vi "GVSGraph Main.vi"() -> ()   [LabVIEW 2013]
uses:
  Control/SplitterBar.ctl
  Control/Graph Main Info Cluster.ctl
  <vilib>/Utility/inputDevices.llb/closeMouse.vi
  GVSNew View Global.vi
  GVSView Global.vi
  <vilib>/Utility/inputDevices.llb/mouseAcquire.vi
  <vilib>/Utility/cursorutil.llb/Set Cursor (Icon Pict).vi
panel:
  in  "bWaitCommand":bool
  in  "Docking Start":bool
  in  "nIDV":i32=10
  in  "pSPRefParent":refnum<vi>
  in  "pVIRefParent":refnum<vi>
  in  "sViewName":string="DataView"
  out "Index":i32
  in  "stop":bool
  out "StateOut":bool
  out "Bar_shadow":bool
  in  "Resize FrontPanel":bool
  in  "Add Top":bool
  in  "Add Left":bool
  out "s2":T1
  out "s30":T1
  out "s29":T1
  out "s28":T1
  out "s27":T1
  out "s26":T1
  out "s25":T1
  in  "Mouse Pos":T2
  in  "ToolbarClicked":bool
  in  "Add Bottom":bool
  in  "activated_idx":i32
  in  "close_panel":bool=TRUE
  in  "Resize_Panels":bool
  in  "splitter_down_flag":bool=TRUE
  in  "spliter_index":i32
  out "s7":T1
  out "s1":T1
  out "s12":T1
  out "s5":T1
  out "s6":T1
  out "s11":T1
  out "s10":T1
  out "s19":T1
  out "s9":T1
  out "s8":T1
  out "s24":T1
  out "s23":T1
  out "s22":T1
  out "s21":T1
  out "s20":T1
  out "s18":T1
  out "s17":T1
  out "s16":T1
  out "s15":T1
  out "s14":T1
  out "s13":T1
  out "s4":T1
  out "s3":T1
  in  "Add Right":bool
types:
  T1 = typedef "SplitterBar.ctl" = bool
  T2 = cluster{"Horizontal":i32, "Vertical":i32, "Scrolling":i32}
  T3 = cluster{"Ctrl Reference":refnum<vi>, "bObjMove":bool, "Position_top":i32, "Position_objtop":i32, "isVertical":bool, "Position_left":i32, "Position_objleft":i32}
  T4 = typedef "Graph Main Info Cluster.ctl" = cluster{"Selected_BarIdx":i32, "Selected_PanelIdx":i32, "Graph Main VIRef":refnum<vi>, "ToolBarClick":bool, "Spliter Ref Array":refnum<vi>[], "Panel Ref Array":refnum<vi>[], "Spliter_matrix":i32[][], "Panel_matrix":i32[][], "child_spliterIdx_matrix":i32[][], "split_pos_matrix":i32[][], "Title State":bool, "sQueueName":string, "Frame nID":i32, "Graph VIRef Array":cluster{"Graph VIRef":refnum<vi>, "Panel Idx":i32, "Frame VIRef":refnum<vi>, "Icon Ring":i32, "Graph Type":string}[], "View Type":string}
  T5 = cluster{"TitlebarActiveColor Graph":u32, "TitlebarActiveColor Graph 2":u32}[]
  T6 = cluster{"sCmdType":string, "nIDView":i32, "sAction":string, "sData":string, "sOption":string, "nData":i32, "nOption":i32, "pVIRef":refnum<vi>, "pSPRef":refnum<vi>, "bWaitRef":refnum<vi>, "Result":variant}
  T7 = cluster{"button 1":bool, "button 2":bool, "button 3":bool, "button 4":bool}
  T8 = typedef "LVRectTypeDef.ctl" = cluster{"Left":i16, "Top":i16, "Right":i16, "Bottom":i16}
  T9 = cluster{"Left":bool, "Top":bool, "Right":bool, "Bottom":bool}
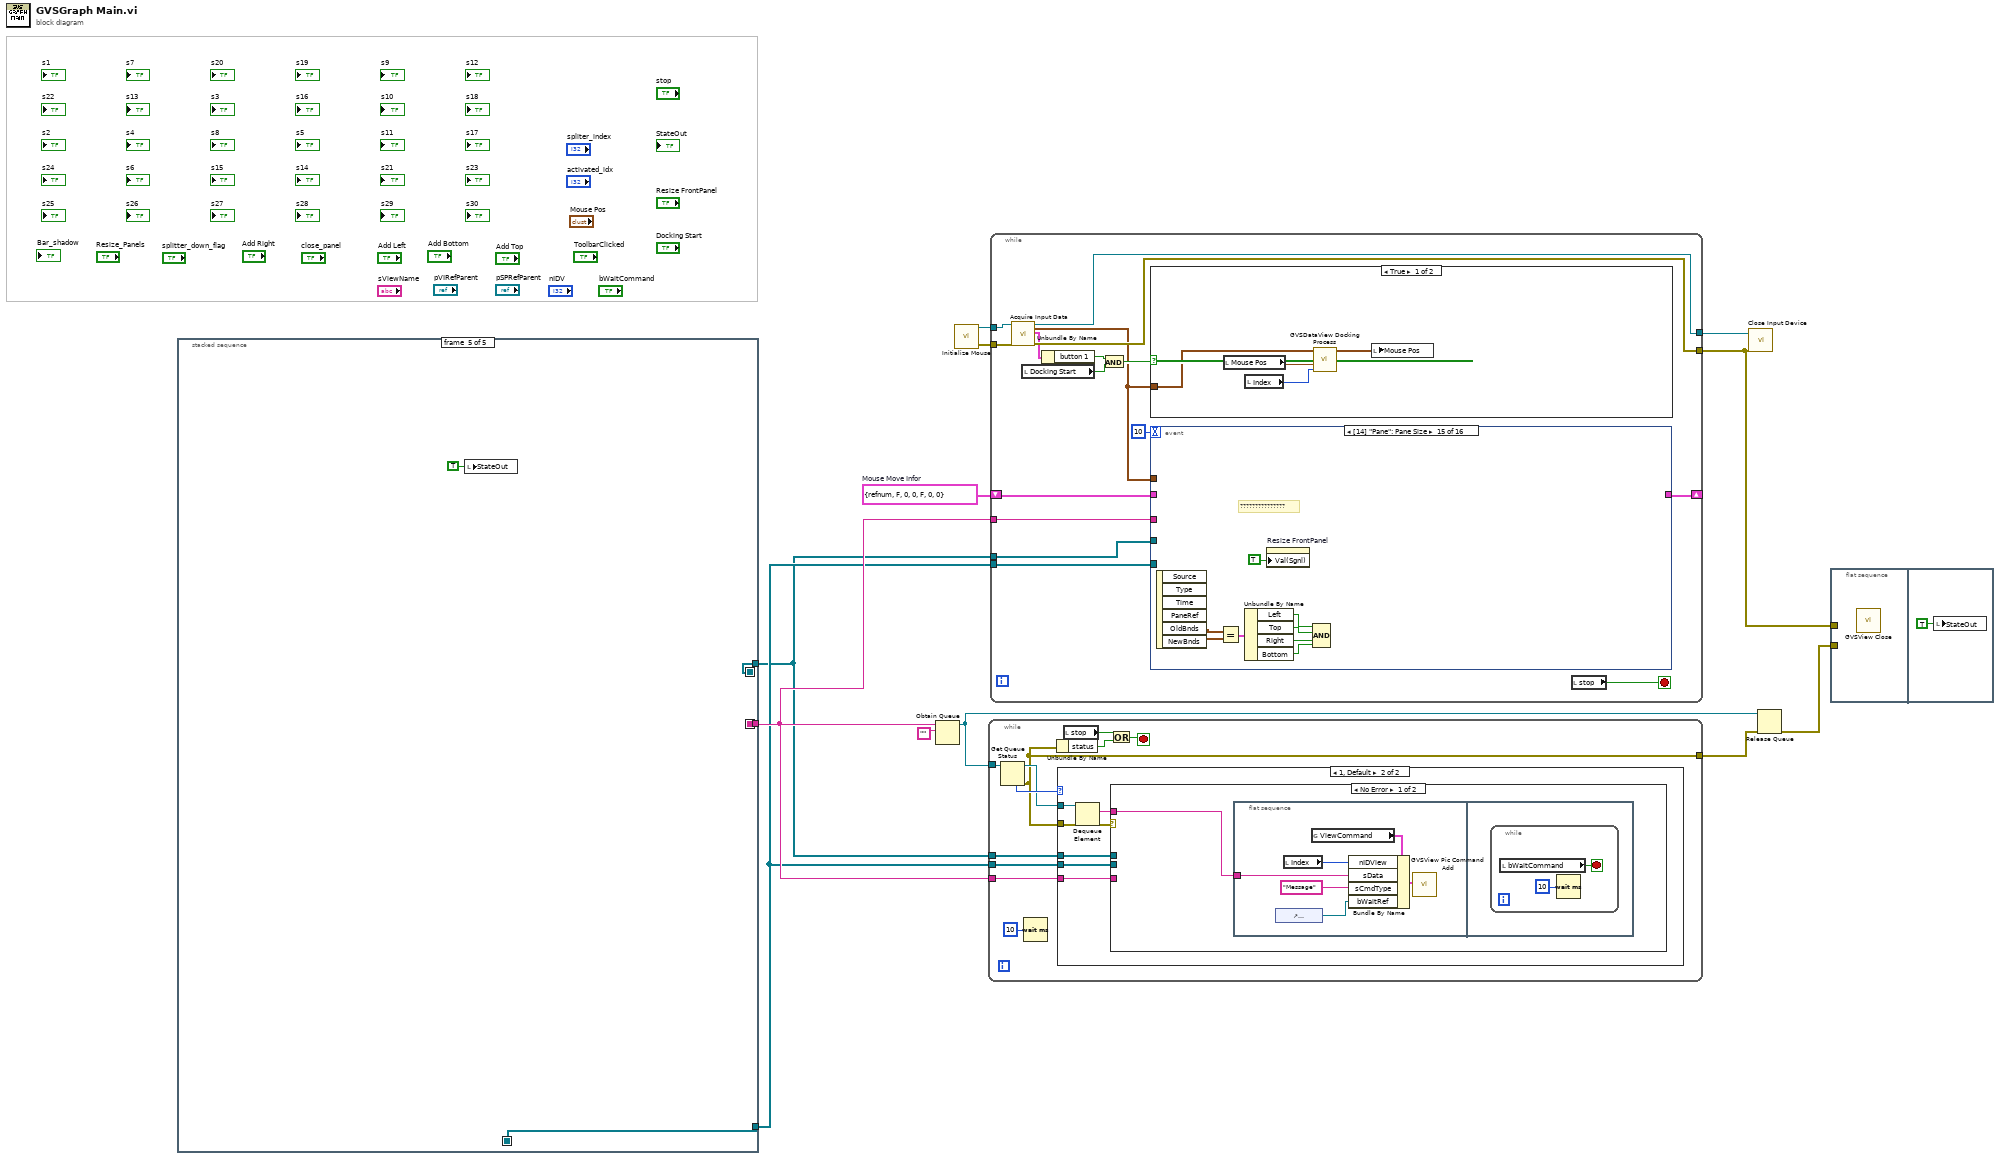
[diagram p0: block diagram]
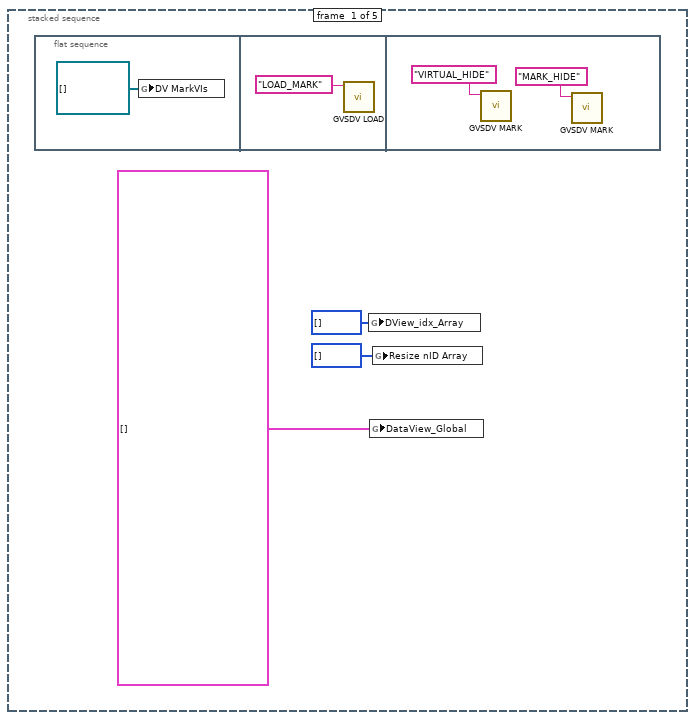
[diagram p2: hidden frame]
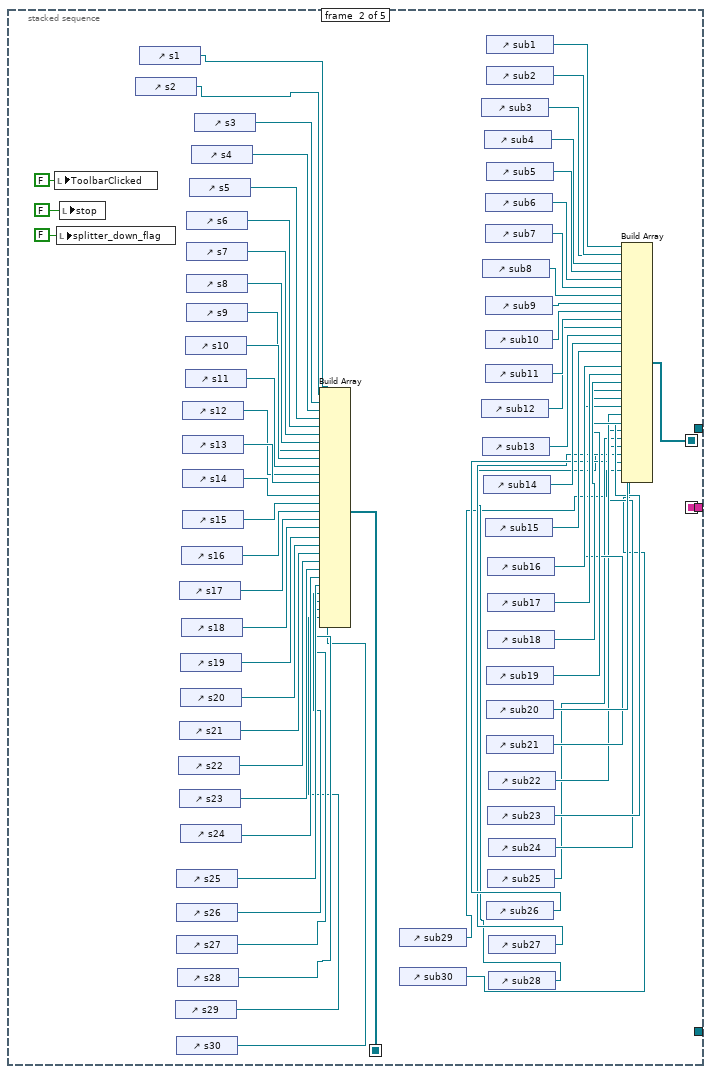
[diagram p3: hidden frame]
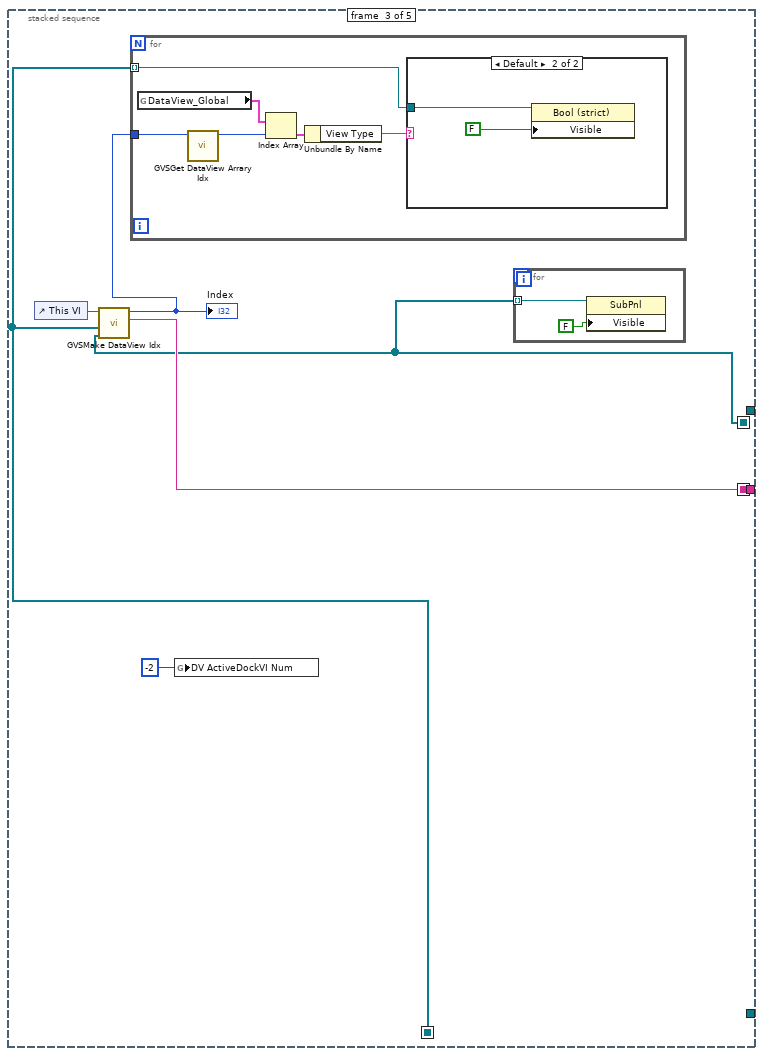
[diagram p4: hidden frame]
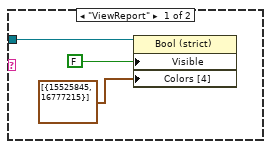
[diagram p5: hidden frame]
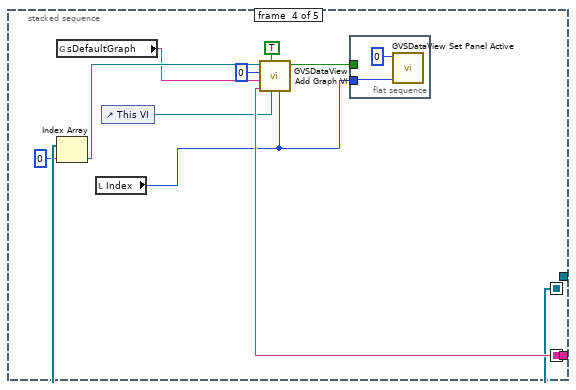
[diagram p6: hidden frame]
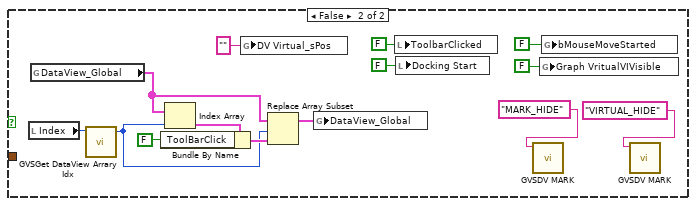
[diagram p9: hidden frame]
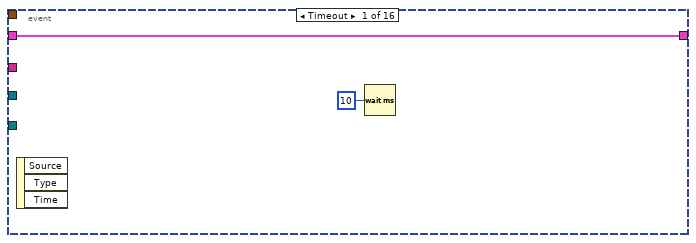
[diagram p10: hidden frame]
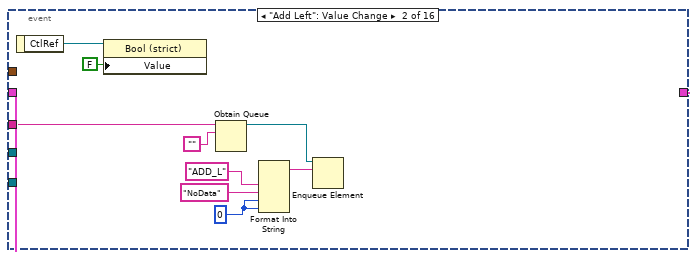
[diagram p11: hidden frame]
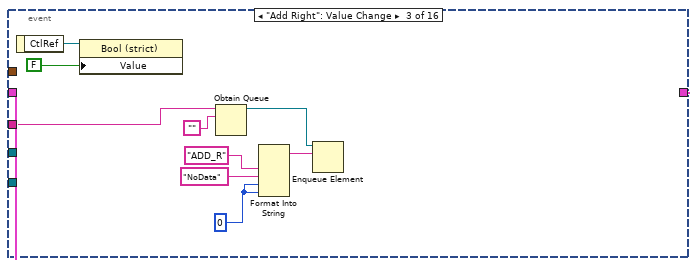
[diagram p12: hidden frame]
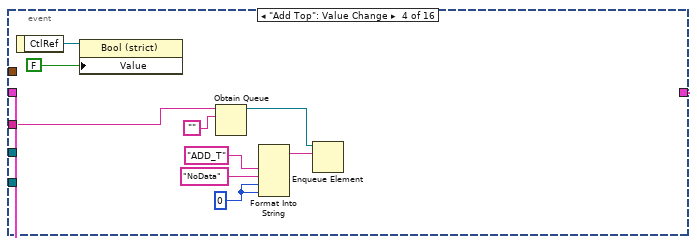
[diagram p13: hidden frame]
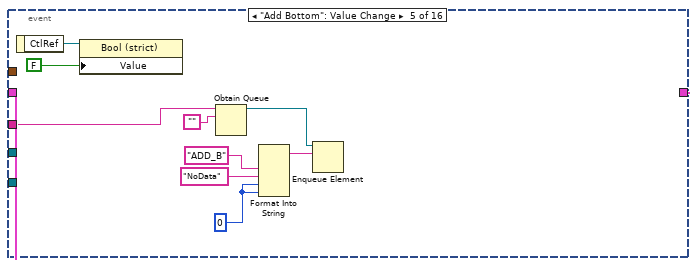
[diagram p14: hidden frame]
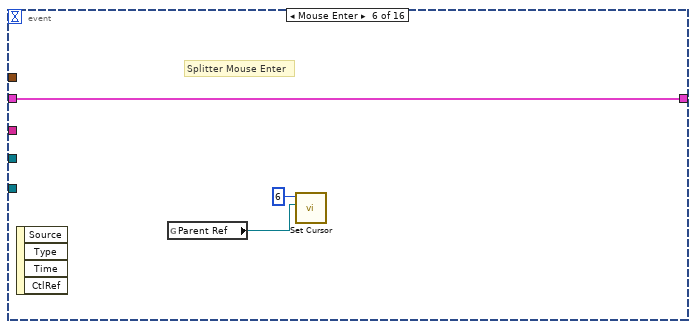
[diagram p15: hidden frame]
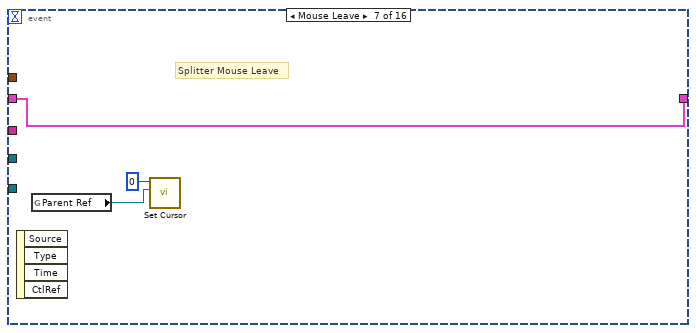
[diagram p16: hidden frame]
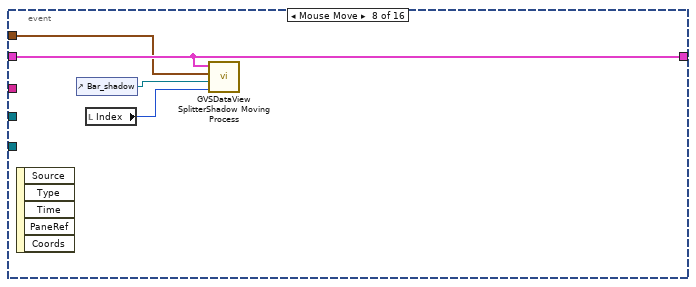
[diagram p17: hidden frame]
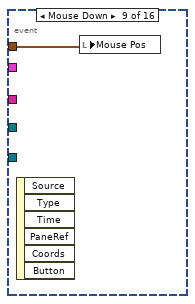
[diagram p18: hidden frame]
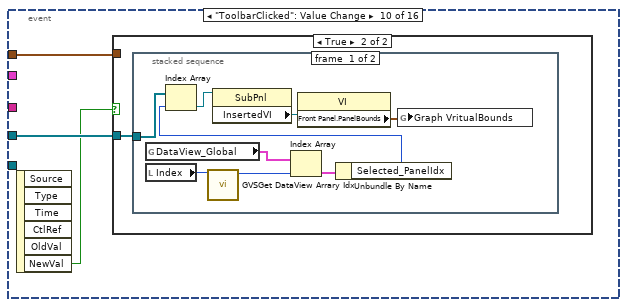
[diagram p19: hidden frame]
diagram:
  w12 = T3 {"Ctrl Reference"=refnum, "bObjMove"=FALSE, "Position_top"=0, "Position_objtop"=0, "isVertical"=FALSE, "Position_left"=0, "Position_objleft"=0}  # Mouse Move Infor
  n1 = stacked-sequence {
    seq-local: [_ w45 _ _ _] -> [_ _ w89 _ w117]
    seq-local: [_ w44 _ _ _] -> [_ _ w85 w112 w116]
    seq-local: [_ _ w88 _ _] -> [_ _ _ w113 _]
    tunnel: [_ _ w88 _ _] -> w4
    tunnel: [_ _ _ _ w117] -> w3
    tunnel: [_ _ _ _ w116] -> w2
    frame #0 {
      n2 = flat-sequence {
        frame #0 {
          n3 = global write "GVSNew View Global.vi" "DV MarkVIs"(refnum<vi>[] [] ("DV MarkVIs")) -> ()
        }
        frame #1 {
          n4 = call "GVSDV LOAD.vi"("sAction"="LOAD_MARK") -> ()  [unwired: 7 in, 4 out]
        }
        frame #2 {
          n5 = call "GVSDV MARK.vi"("sAction"="VIRTUAL_HIDE") -> ()  [unwired: 9 in, 1 out]
          n6 = call "GVSDV MARK.vi"("sAction"="MARK_HIDE") -> ()  [unwired: 9 in, 1 out]
        }
      }
      n7 = global write "GVSNew View Global.vi" "DView_idx_Array"(i32[] [] ("DView_idx_Array")) -> ()
      n8 = global write "GVSNew View Global.vi" "DataView_Global"(T4[] [] ("DataView_Global")) -> ()
      n9 = global write "GVSNew View Global.vi" "Resize nID Array"(i32[] [] ("Resize nID Array")) -> ()
    }
    frame #1 {
      n10 = local write "ToolbarClicked"(FALSE ("ToolbarClicked")) -> ()
      n11 = local write "splitter_down_flag"(FALSE ("m_down_flag")) -> ()
      n12 = local write "stop"(FALSE ("stop")) -> ()
      n13 = control-ref of="s2"() -> (w20:refnum<vi>)
      n14 = control-ref of="s1"() -> (w21:refnum<vi>)
      n15 = control-ref of="s29"() -> (w26:refnum<vi>)
      n16 = control-ref of="s25"() -> (w30:refnum<vi>)
      n17 = control-ref of="s26"() -> (w29:refnum<vi>)
      n18 = control-ref of="s27"() -> (w28:refnum<vi>)
      n19 = control-ref of="s30"() -> (w25:refnum<vi>)
      n20 = control-ref of="s28"() -> (w27:refnum<vi>)
      n21 = control-ref of="s22"() -> (w66:refnum<vi>)
      n22 = control-ref of="s17"() -> (w61:refnum<vi>)
      n23 = control-ref of="s21"() -> (w65:refnum<vi>)
      n24 = control-ref of="s23"() -> (w67:refnum<vi>)
      n25 = control-ref of="s19"() -> (w63:refnum<vi>)
      n26 = control-ref of="s20"() -> (w64:refnum<vi>)
      n27 = control-ref of="s24"() -> (w68:refnum<vi>)
      n28 = control-ref of="s16"() -> (w60:refnum<vi>)
      n29 = control-ref of="s18"() -> (w62:refnum<vi>)
      n30 = control-ref of="s12"() -> (w56:refnum<vi>)
      n31 = control-ref of="s13"() -> (w57:refnum<vi>)
      n32 = control-ref of="s14"() -> (w58:refnum<vi>)
      n33 = control-ref of="s15"() -> (w59:refnum<vi>)
      n34 = control-ref of="s10"() -> (w54:refnum<vi>)
      n35 = control-ref of="s11"() -> (w55:refnum<vi>)
      n36 = control-ref of="s6"() -> (w50:refnum<vi>)
      n37 = control-ref of="s7"() -> (w51:refnum<vi>)
      n38 = control-ref of="s8"() -> (w52:refnum<vi>)
      n39 = control-ref of="s9"() -> (w53:refnum<vi>)
      n40 = control-ref of="s5"() -> (w49:refnum<vi>)
      n41 = control-ref of="s4"() -> (w48:refnum<vi>)
      n42 = control-ref of="s3"() -> (w47:refnum<vi>)
      n43 = Build Array(w21, w20, w47, w48, w49, w50, w51, w52, w53, w54, w55, w56, w57, w58, w59, w60, w61, w62, w63, w64, w65, w66, w67, w68, w30, w29, w28, w27, w26, w25) -> (w45:refnum<vi>[])
      n44 = control-ref of="sub29"() -> (w32:refnum<vi>)
      n45 = control-ref of="sub30"() -> (w31:refnum<vi>)
      n46 = control-ref of="sub3"() -> (w22:refnum<vi>)
      n47 = control-ref of="sub12"() -> (w75:refnum<vi>)
      n48 = control-ref of="sub8"() -> (w78:refnum<vi>)
      n49 = control-ref of="sub13"() -> (w74:refnum<vi>)
      n50 = control-ref of="sub14"() -> (w73:refnum<vi>)
      n51 = control-ref of="sub4"() -> (w82:refnum<vi>)
      n52 = control-ref of="sub6"() -> (w80:refnum<vi>)
      n53 = control-ref of="sub7"() -> (w79:refnum<vi>)
      n54 = control-ref of="sub9"() -> (w77:refnum<vi>)
      n55 = control-ref of="sub10"() -> (w69:refnum<vi>)
      n56 = control-ref of="sub11"() -> (w76:refnum<vi>)
      n57 = control-ref of="sub15"() -> (w72:refnum<vi>)
      n58 = control-ref of="sub1"() -> (w84:refnum<vi>)
      n59 = control-ref of="sub2"() -> (w83:refnum<vi>)
      n60 = control-ref of="sub5"() -> (w81:refnum<vi>)
      n61 = control-ref of="sub19"() -> (w42:refnum<vi>)
      n62 = control-ref of="sub20"() -> (w41:refnum<vi>)
      n63 = control-ref of="sub21"() -> (w40:refnum<vi>)
      n64 = control-ref of="sub26"() -> (w35:refnum<vi>)
      n65 = control-ref of="sub16"() -> (w71:refnum<vi>)
      n66 = control-ref of="sub17"() -> (w70:refnum<vi>)
      n67 = control-ref of="sub18"() -> (w43:refnum<vi>)
      n68 = control-ref of="sub23"() -> (w38:refnum<vi>)
      n69 = control-ref of="sub25"() -> (w36:refnum<vi>)
      n70 = control-ref of="sub22"() -> (w39:refnum<vi>)
      n71 = control-ref of="sub24"() -> (w37:refnum<vi>)
      n72 = control-ref of="sub27"() -> (w34:refnum<vi>)
      n73 = control-ref of="sub28"() -> (w33:refnum<vi>)
      n74 = Build Array(w84, w83, w22, w82, w81, w80, w79, w78, w77, w69, w76, w75, w74, w73, w72, w71, w70, w43, w42, w41, w40, w39, w38, w37, w36, w35, w34, w33, w32, w31) -> (w44:refnum<vi>[])
    }
    frame #2 {
      n75 = control-ref of="This VI"() -> (w90:refnum<vi>)
      n76 = call "GVSMake DataView Idx.vi"("Panel Ref Array"=w85, "Spliter Ref Array"=w89, "VI Ref"=w90) -> ("sQueueName Out"=w88:string, "New DataView Idx"=w87:i32)  [unwired: 7 in]
      "Index" <- w87
      n77 = for {
        tunnel: w89 -> [w98] mode=indexing
        tunnel: w87 -> [w94]
        n78 = global read "GVSNew View Global.vi" "DataView_Global"() -> (w97:T4[])
        n79 = call "GVSGet DataView Arrary Idx.vi"("DataView Idx In"=w94) -> ("DataView Arrary Idx out"=w95:i32)  [unwired: 10 in]
        n80 = Index Array(array=w97, index=w95) -> (element=w96:T4)
        n81 = Unbundle By Name(w96) -> ("View Type"=w93:string)
        n82 = case shown="Default" w93 {
          tunnel: w98 -> [w100 w102]
          frame "ViewReport" {
            n83 = property class="Bool (strict)"(reference=w100, "Visible"=FALSE, "Colors [4]"=T5 [{"TitlebarActiveColor Graph"=15525845, "TitlebarActiveColor Graph 2"=16777215}]) -> ()  [unwired: 1 in, 2 out]
          }
          frame Default {
            n84 = property class="Bool (strict)"(reference=w102, "Visible"=FALSE) -> ()  [unwired: 1 in, 2 out]
          }
        }
      }
      n85 = global write "GVSNew View Global.vi" "DV ActiveDockVI Num"(-2 ("DV ActiveDockVI Num")) -> ()
      n86 = for {
        tunnel: w85 -> [w91] mode=indexing
        n87 = property class="SubPnl"(reference=w91, "Visible"=FALSE) -> ()  [unwired: 1 in, 2 out]
      }
    }
    frame #3 {
      n88 = global read "GVSView Global.vi" "sDefaultGraph"() -> (w107:string)
      n89 = Index Array(array=w112, index=0) -> (element=w110:refnum<vi>)
      n90 = local read "Index"() -> (w104:i32)
      n91 = control-ref of="This VI"() -> (w106:refnum<vi>)
      n92 = call "GVSDataView Add Graph VI.vi"("DataView Idx"=w104, "Graph Main VIRef In"=w106, "isFirstPanel"=TRUE, "Queue Name"=w113, "GraphType"=w107, "panel_index"=0, "Panel Ref In"=w110) -> ("bResult"=w105:bool)  [unwired: 4 in]
      n93 = flat-sequence {
        tunnel: w104 -> [w115]
        tunnel: w105 -> [_]
        frame #0 {
          n94 = call "GVSDataView Set Panel Active.vi"("DataView Index"=w115, "Selected Panel Idx In"=0) -> ()  [unwired: 10 in]
        }
      }
    }
    frame #4 {
      n95 = local write "StateOut"(TRUE ("StateOut")) -> ()
    }
  }
  n96 = Obtain Queue(name (unnamed)=w4, element data type="") -> (queue out=w10:refnum<queue>)  [unwired: 3 in, 2 out]
  n97 = call <vilib>:"Initialize Mouse.vi"() -> ("error out"=w8:errorcluster, "device ID"=w9:refnum<k1>)  [unwired: 10 in]
  n98 = while {
    tunnel: w10 -> [w128]
    tunnel: w3 -> [w125]
    tunnel: w2 -> [w124]
    tunnel: [w123] -> w6
    tunnel: w4 -> [w119]
    stop <- w120 stop-if-true
    n99 = Get Queue Status(queue=w128) -> (queue out=w126:refnum<queue>, error out=w123:errorcluster, # elements in queue=w127:i32)  [unwired: 2 in, 5 out]
    n100 = Wait (ms)(milliseconds to wait=u32 10) -> ()  [unwired: 1 out]
    n101 = Unbundle By Name(w123) -> ("status"=w122:bool)
    n102 = case shown="1, Default" w127 {
      tunnel: w123 -> [_ w132]
      tunnel: w126 -> [_ w136]
      tunnel: w125 -> [_ w134]
      tunnel: w124 -> [_ w133]
      tunnel: w119 -> [_ w130]
      frame 0 {
      }
      frame 1, Default {
        n103 = Dequeue Element(queue=w136, error in (no error)=w132) -> (element=w135:string, error out=w131:errorcluster)  [unwired: 1 in, 2 out]
        n104 = case shown="No Error" w131 {
          tunnel: w135 -> [w137 _]
          tunnel: w134 -> [_ _]
          tunnel: w133 -> [_ _]
          tunnel: w130 -> [_ _]
          frame No Error {
            n105 = flat-sequence {
              tunnel: w137 -> [w143]
              frame #0 {
                n106 = control-ref of="bWaitCommand"() -> (w140:refnum<vi>)
                n107 = local read "Index"() -> (w138:i32)
                n108 = global read "GVSView Global.vi" "ViewCommand"() -> (w139:T6)
                n109 = Bundle By Name(cluster=w139, "nIDView"=w138, "sData"=w143, "sCmdType"="Message" ("sAction"), "bWaitRef"=w140) -> (w141:T6)
                n110 = call "GVSView Pic Command Add.vi"("cCommand"=w141) -> ()  [unwired: 11 in]
              }
              frame #1 {
                n111 = while {
                  stop <- w145 stop-if-true
                  n112 = local read "bWaitCommand"() -> (w145:bool)
                  n113 = Wait (ms)(milliseconds to wait=u32 10) -> ()  [unwired: 1 out]
                }
              }
            }
          }
          frame Error {
          }
        }
      }
    }
    n114 = local read "stop"() -> (w121:bool)
    n115 = Or(x=w121, y=w122) -> (x .or. y?=w120:bool)
  }
  n116 = while {
    tunnel: w2 -> [w148]
    shift-right: [w159] -> _
    shift-left: w12 -> [w161]
    tunnel: w3 -> [w160]
    tunnel: w4 -> [w158]
    tunnel: w9 -> [w157]
    tunnel: w8 -> [w146]
    tunnel: [w156] -> w7
    tunnel: [w155] -> w1
    stop <- w147 stop-if-true
    n117 = call-poly <vilib>:"Acquire Input Data.vi"("device ID"=w157, "error in (no error)"=w146) -> ("device ID"=w156:refnum<k1>, "axis info"=w149:T2, "button info"=w154:T7, "error out"=w155:errorcluster)  [unwired: 14 in]
    n118 = local read "Docking Start"() -> (w152:bool)
    n119 = Unbundle By Name(w154) -> ("button 1"=w151:bool)
    n120 = And(x=w151, y=w152) -> (x .and. y?=w150:bool)
    n121 = event shown="[14] \"Pane\": Pane Size" {
      selector: _ -> [_ _ _ _ _ _ _ _ _ _ _ _ _ _ _ _]
      dyn-events: _ -> [_ _ _ _ _ _ _ _ _ _ _ _ _ _ _ _]
      timeout: 10 -> [_ _ _ _ _ _ _ _ _ _ _ _ _ _ _ _]
      tunnel: w148 -> [_ _ _ _ _ _ _ _ _ w234 _ _ _ _ _ _]
      tunnel: w161 -> [w180 w189 w199 w209 w219 w224 w227 w231 _ _ w249 w256 w265 w281 _ _]
      tunnel: [w180 w189 w199 w209 w219 w224 w227 w231 _ _ w248 w258 w267 w282 _ _] -> w159
      tunnel: w160 -> [_ _ _ _ _ _ _ _ _ _ _ _ _ _ _ _]
      tunnel: w158 -> [_ w182 w192 w202 w212 _ _ _ _ _ _ _ _ w274 _ _]
      tunnel: w149 -> [_ _ _ _ _ _ _ w230 w232 w235 w250 _ _ _ _ _]
      event Timeout {
        n122 = event-data() -> ()  [unwired: 1 in, 3 out]
        n123 = Wait (ms)(milliseconds to wait=u32 10) -> ()  [unwired: 1 out]
      }
      event "Add Left": Value Change {
        w183 = 0 ("input 3")
        n124 = event-data() -> ("CtlRef"=w191:refnum<vi>)  [unwired: 1 in]
        n125 = property class="Bool (strict)"(reference=w191, "Value"=FALSE) -> ()  [unwired: 1 in, 2 out]
        n126 = Obtain Queue(name (unnamed)=w182, element data type="") -> (queue out=w185:refnum<queue>)  [unwired: 3 in, 2 out]
        n127 = Format Into String("ADD_L" ("input 1"), "NoData" ("input 2"), w183, w183) -> (resulting string=w184:string)  [unwired: 3 in, 1 out]
        n128 = Enqueue Element(queue=w185, element=w184) -> ()  [unwired: 1 in, 4 out]
      }
      event "Add Right": Value Change {
        w193 = 0 ("input 3")
        n129 = event-data() -> ("CtlRef"=w201:refnum<vi>)  [unwired: 1 in]
        n130 = property class="Bool (strict)"(reference=w201, "Value"=FALSE) -> ()  [unwired: 1 in, 2 out]
        n131 = Obtain Queue(name (unnamed)=w192, element data type="") -> (queue out=w195:refnum<queue>)  [unwired: 3 in, 2 out]
        n132 = Format Into String("ADD_R" ("input 1"), "NoData" ("input 2"), w193, w193) -> (resulting string=w194:string)  [unwired: 3 in, 1 out]
        n133 = Enqueue Element(queue=w195, element=w194) -> ()  [unwired: 1 in, 4 out]
      }
      event "Add Top": Value Change {
        w203 = 0 ("input 3")
        n134 = event-data() -> ("CtlRef"=w211:refnum<vi>)  [unwired: 1 in]
        n135 = property class="Bool (strict)"(reference=w211, "Value"=FALSE) -> ()  [unwired: 1 in, 2 out]
        n136 = Obtain Queue(name (unnamed)=w202, element data type="") -> (queue out=w205:refnum<queue>)  [unwired: 3 in, 2 out]
        n137 = Format Into String("ADD_T" ("input 1"), "NoData" ("input 2"), w203, w203) -> (resulting string=w204:string)  [unwired: 3 in, 1 out]
        n138 = Enqueue Element(queue=w205, element=w204) -> ()  [unwired: 1 in, 4 out]
      }
      event "Add Bottom": Value Change {
        w213 = 0 ("input 3")
        n139 = event-data() -> ("CtlRef"=w221:refnum<vi>)  [unwired: 1 in]
        n140 = property class="Bool (strict)"(reference=w221, "Value"=FALSE) -> ()  [unwired: 1 in, 2 out]
        n141 = Obtain Queue(name (unnamed)=w212, element data type="") -> (queue out=w215:refnum<queue>)  [unwired: 3 in, 2 out]
        n142 = Format Into String("ADD_B" ("input 1"), "NoData" ("input 2"), w213, w213) -> (resulting string=w214:string)  [unwired: 3 in, 1 out]
        n143 = Enqueue Element(queue=w215, element=w214) -> ()  [unwired: 1 in, 4 out]
      }
      event Mouse Enter {
        # "Splitter Mouse Enter"
        n144 = event-data() -> ()  [unwired: 1 in, 4 out]
        n145 = global read "GVSNew View Global.vi" "Parent Ref"() -> (w222:refnum<vi>)
        n146 = call-poly <vilib>:"Set Cursor.vi"("VI reference (current VI)"=w222, "icon"=u16 6) -> ()  [unwired: 1 in, 9 out]
      }
      event Mouse Leave {
        # "Splitter Mouse Leave"
        n147 = event-data() -> ()  [unwired: 1 in, 4 out]
        n148 = global read "GVSNew View Global.vi" "Parent Ref"() -> (w225:refnum<vi>)
        n149 = call-poly <vilib>:"Set Cursor.vi"("VI reference (current VI)"=w225, "icon"=u16 0) -> ()  [unwired: 1 in, 9 out]
      }
      event Mouse Move {
        n150 = event-data() -> ()  [unwired: 1 in, 5 out]
        n151 = control-ref of="Bar_shadow"() -> (w229:refnum<vi>)
        n152 = local read "Index"() -> (w228:i32)
        n153 = call "GVSDataView SplitterShadow Moving Process.vi"("DataView Index"=w228, "Bar_shadow ref"=w229, "Mouse Pos"=w230, "SpliterMoveInfo"=w231) -> ()  [unwired: 8 in]
      }
      event Mouse Down {
        n154 = event-data() -> ()  [unwired: 1 in, 6 out]
        n155 = local write "Mouse Pos"(w232) -> ()
      }
      event "ToolbarClicked": Value Change {
        n156 = event-data() -> ("NewVal"=w233:bool)  [unwired: 1 in, 5 out]
        n157 = case shown="True" w233 {
          tunnel: w235 -> [_ _]
          tunnel: w234 -> [_ w236]
          frame False {
          }
          frame True {
            n158 = stacked-sequence {
              tunnel: w236 -> [w243 _]
              frame #0 {
                n159 = global read "GVSNew View Global.vi" "DataView_Global"() -> (w245:T4[])
                n160 = local read "Index"() -> (w238:i32)
                n161 = call "GVSGet DataView Arrary Idx.vi"("DataView Idx In"=w238) -> ("DataView Arrary Idx out"=w237:i32)  [unwired: 10 in]
                n162 = Index Array(array=w245, index=w237) -> (element=w244:T4)
                n163 = Unbundle By Name(w244) -> ("Selected_PanelIdx"=w242:i32)
                n164 = Index Array(array=w243, index=w242) -> (element=w241:refnum<vi>)
                n165 = property class="SubPnl"(reference=w241) -> ("InsertedVI"=w240:refnum<vi>)  [unwired: 1 in, 2 out]
                n166 = property class="VI"(reference=w240) -> ("Front Panel.PanelBounds"=w239:T8)  [unwired: 1 in, 2 out]
                n167 = global write "GVSNew View Global.vi" "Graph VritualBounds"(w239) -> ()
              }
              frame #1 {
                n168 = local write "Docking Start"(TRUE ("Docking Start")) -> ()
              }
            }
          }
        }
      }
      event Mouse Down {
        # "Splitter Mouse down"
        n169 = event-data() -> ("CtlRef"=w247:refnum<vi>)  [unwired: 1 in, 5 out]
        n170 = control-ref of="Bar_shadow"() -> (w253:refnum<vi>)
        n171 = local read "Index"() -> (w251:i32)
        n172 = call "GVSDataView Splitter MDown Process.vi"("DataView Index"=w251, "Selected Spliter Ref"=w247, "Bar_shadow ref"=w253, "Mouse Pos"=w250, "SpliterMove Info"=w249) -> ("SpliterMove Out"=w248:T3)  [unwired: 6 in]
        n173 = local write "splitter_down_flag"(TRUE ("m_down_flag")) -> ()
      }
      event Mouse Up {
        n174 = event-data() -> ()  [unwired: 1 in, 8 out]
        n175 = local read "splitter_down_flag"() -> (w257:bool)
        n176 = Bundle By Name(cluster=w256, "bObjMove"=FALSE ("객체이동")) -> (w258:T3)
        n177 = case shown="True" w257 {
          frame False {
          }
          frame True {
            n178 = local write "splitter_down_flag"(FALSE ("m_down_flag")) -> ()
            n179 = property on="Resize_Panels" class="Bool (strict)"("Val(Sgnl)"=TRUE ("Value (Signaling)")) -> ()  [unwired: 2 in, 2 out]
            n180 = local write "close_panel"(FALSE ("close_panel")) -> ()
          }
        }
        n181 = global read "GVSNew View Global.vi" "Parent Ref"() -> (w254:refnum<vi>)
        n182 = call-poly <vilib>:"Set Cursor.vi"("VI reference (current VI)"=w254, "icon"=u16 0) -> ()  [unwired: 1 in, 9 out]
      }
      event Mouse Leave {
        n183 = event-data() -> ()  [unwired: 1 in, 4 out]
        n184 = local read "splitter_down_flag"() -> (w266:bool)
        n185 = Bundle By Name(cluster=w265, "bObjMove"=FALSE ("객체이동")) -> (w267:T3)
        n186 = case shown="True" w266 {
          frame False {
          }
          frame True {
            n187 = local write "splitter_down_flag"(FALSE ("m_down_flag")) -> ()
            n188 = local write "close_panel"(FALSE ("close_panel")) -> ()
            n189 = property on="Resize_Panels" class="Bool (strict)"("Val(Sgnl)"=TRUE ("Value (Signaling)")) -> ()  [unwired: 2 in, 2 out]
          }
        }
        n190 = global read "GVSNew View Global.vi" "Parent Ref"() -> (w263:refnum<vi>)
        n191 = call-poly <vilib>:"Set Cursor.vi"("VI reference (current VI)"=w263, "icon"=u16 0) -> ()  [unwired: 1 in, 9 out]
      }
      event "Resize_Panels": Value Change {
        n192 = event-data() -> ()  [unwired: 1 in, 6 out]
        n193 = Bundle By Name(cluster=w281, "bObjMove"=FALSE ("객체이동")) -> (w282:T3)
        n194 = local read "Index"() -> (w273:i32)
        n195 = Obtain Queue(name (unnamed)=w274, element data type="") -> (queue out=w278:refnum<queue>)  [unwired: 3 in, 2 out]
        n196 = Format Into String("GRAPH_MAIN_SUBPANEL_RESIZE" ("input 1"), "NoData" ("input 2"), 0 ("input 3"), w273) -> (resulting string=w279:string)  [unwired: 3 in, 1 out]
        n197 = local write "Resize_Panels"(FALSE ("Resize_Panels")) -> ()
        n198 = Enqueue Element(queue=w278, element=w279) -> ()  [unwired: 1 in, 4 out]
        n199 = disable-structure shown="Disabled" {
          frame Disabled {
            n200 = call-poly <vilib>:"Set Cursor.vi"("icon"=u16 1) -> ()  [unwired: 2 in, 9 out]
          }
          frame Enabled {
          }
        }
      }
      event Pane Size {
        # "???????????????"
        n201 = event-data() -> ("OldBnds"=w292:T8, "NewBnds"=w291:T8)  [unwired: 1 in, 4 out]
        n202 = Equal?(x=w292, y=w291) -> (x = y?=w290:T9)
        n203 = Unbundle By Name(w290) -> ("Left"=w289:bool, "Top"=w288:bool, "Right"=w287:bool, "Bottom"=w286:bool)
        n204 = property on="Resize FrontPanel" class="Bool (strict)"("Val(Sgnl)"=TRUE ("Value (Signaling)")) -> ()  [unwired: 2 in, 2 out]
        n205 = Compound Arithmetic op=AND(w289, w288, w287, w286) -> ()  [unwired: 1 out]
      }
      event "Resize FrontPanel": Value Change {
        n206 = event-data() -> ()  [unwired: 1 in, 6 out]
        n207 = control-ref of="This VI"() -> (w294:refnum<vi>)
        n208 = local read "Index"() -> (w293:i32)
        n209 = local write "Resize FrontPanel"(FALSE ("Resize FrontPanel")) -> ()
        n210 = call "GVSDataView Pane Resize Proc.vi"("DataView Index"=w293, "VI Ref"=w294) -> ()  [unwired: 10 in]
      }
    }
    n211 = case shown="True" w150 {
      tunnel: w149 -> [w165 _]
      frame True {
        n212 = local read "Mouse Pos"() -> (w164:T2)
        n213 = local read "Index"() -> (w162:i32)
        n214 = call "GVSDataView Docking Process.vi"("DataView Index"=w162, "Start Pos"=w164, "Mouse Pos"=w165) -> ("StartPositin Out"=w163:T2)  [unwired: 8 in]
        n215 = local write "Mouse Pos"(w163) -> ()
      }
      frame False {
        n216 = local read "Index"() -> (w179:i32)
        n217 = global read "GVSNew View Global.vi" "DataView_Global"() -> (w174:T4[])
        n218 = call "GVSGet DataView Arrary Idx.vi"("DataView Idx In"=w179) -> ("DataView Arrary Idx out"=w169:i32)  [unwired: 10 in]
        n219 = Index Array(array=w174, index=w169) -> (element=w177:T4)
        n220 = Bundle By Name(cluster=w177, "ToolBarClick"=FALSE) -> (w176:T4)
        n221 = global write "GVSNew View Global.vi" "DV Virtual_sPos"("" ("DV Virtual_sPos")) -> ()
        n222 = Replace Array Subset(array=w174, new element=w176, index=w169) -> (w178:T4[])
        n223 = global write "GVSNew View Global.vi" "DataView_Global"(w178) -> ()
        n224 = local write "ToolbarClicked"(FALSE ("ToolbarClicked")) -> ()
        n225 = local write "Docking Start"(FALSE ("Docking Start")) -> ()
        n226 = call "GVSDV MARK.vi"("sAction"="MARK_HIDE") -> ()  [unwired: 9 in, 1 out]
        n227 = global write "GVSNew View Global.vi" "Graph VritualVIVisible"(FALSE ("VritualVIVisible")) -> ()
        n228 = global write "GVSNew View Global.vi" "bMouseMoveStarted"(FALSE ("VritualVIVisible")) -> ()
        n229 = call "GVSDV MARK.vi"("sAction"="VIRTUAL_HIDE") -> ()  [unwired: 9 in, 1 out]
      }
    }
    n230 = local read "stop"() -> (w147:bool)
  }
  n231 = call-poly <vilib>:"Close Input Device.vi"("error in (no error)"=w1, "device ID"=w7) -> ()  [unwired: 8 in, 1 out]
  n232 = Release Queue(queue=w10, error in (no error)=w6) -> (error out=w5:errorcluster)  [unwired: 1 in, 2 out]
  n233 = flat-sequence {
    tunnel: w5 -> [_]
    tunnel: w1 -> [_]
    frame #0 {
      n234 = call "GVSView Close.vi"() -> ()  [unwired: 12 in]
    }
    frame #1 {
      n235 = local write "StateOut"(TRUE ("StateOut")) -> ()
    }
  }
